vi "GlobalVariables.vi"() -> ()   [LabVIEW 2020]
panel:
  out "Abr_mov":bool
  in  "Rate_Test":dbl
  out "Disp_ON":bool
  in  "Valor_sensor":dbl
  in  "Disp_Valido":dbl
  in  "pwm_shot":dbl
  out "POVs":i16[](array[numeric])
  out "Axes":dbl[](array[numeric])
  out "Buttons":bool[](array[boolean])
  in  "Disparo_Max":dbl
  out "ValidTarget":bool
  in  "Ty":dbl
  in  "Tx":dbl
  out "Buttons_axes":bool
  in  "Dist_Braco":dbl
  in  "Pos_Braco":dbl
  out "Aim_Lock":bool
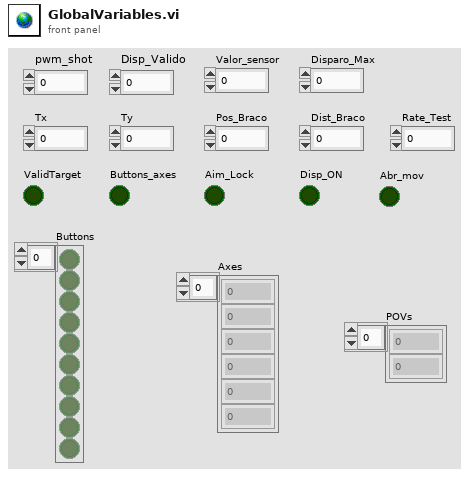
[diagram p1: front panel]
diagram:
